vi "Word Finder.vi"() -> ()   [LabVIEW 2023]
uses:
  af6e6935-e207-d649-a71b-7505053b652b.vi
panel:
  out "msg":string
  out "words":string[](array[string])
  in  "file":path=path "Gettysburg.txt"
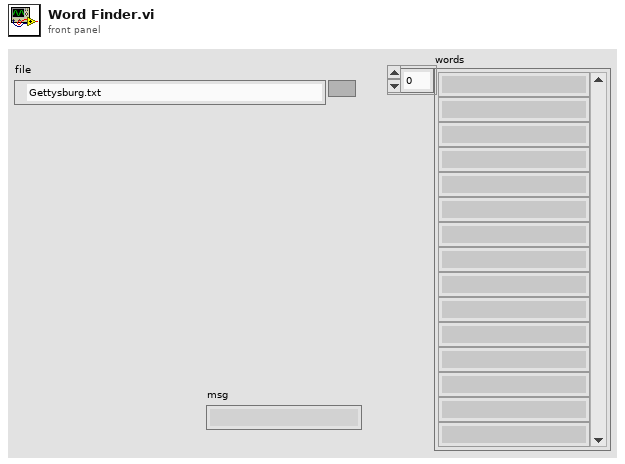
[diagram p1: front panel]
types:
  T1 = enum16{"_Quit_", "Init", "Space", "Word", "Error", "Done"}
  T2 = enum16{"_Quit_", "Init", "Space", "Word", "Error", "Done"}[]
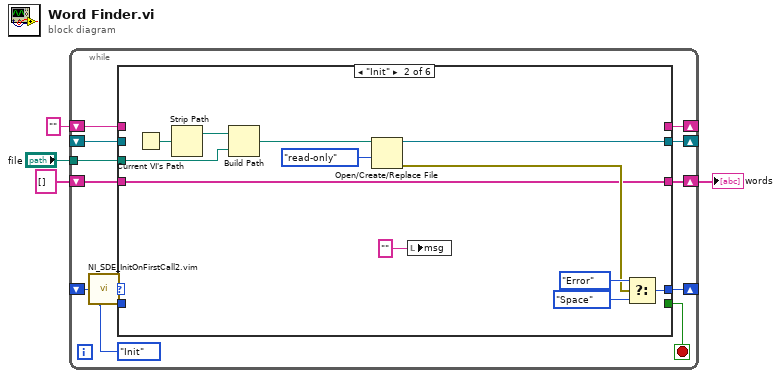
[diagram p0: block diagram]
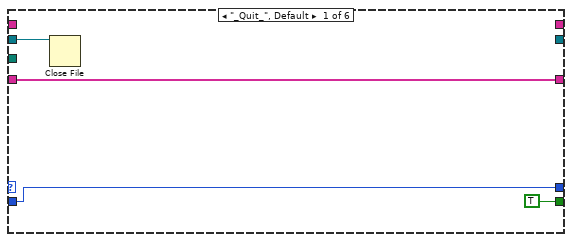
[diagram p2: hidden frame]
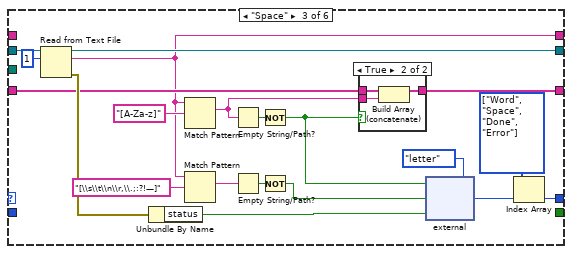
[diagram p3: hidden frame]
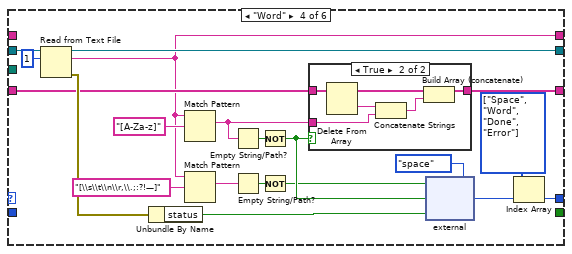
[diagram p5: hidden frame]
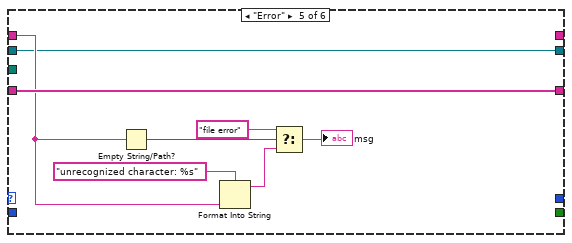
[diagram p7: hidden frame]
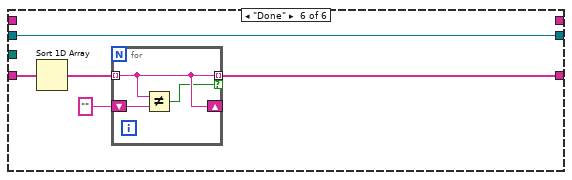
[diagram p8: hidden frame]
diagram:
  n1 = while {
    shift-right: [w12] -> w3
    shift-left: string[] [] -> [w11]
    tunnel: "file" -> [w14]
    shift-right: [w13] -> _
    shift-left: _ -> [w10]
    shift-right: [w9] -> _
    shift-left: "" -> [w8]
    shift-right: [w7] -> _
    shift-left: _ -> [w6]
    stop <- w16 stop-if-true
    w15 = T1."Init"
    n2 = call "NI_SDE_InitOnFirstCall2.vim"("input"=w6, "master enum"=w15) -> ("output enum"=w5:T1)  [unwired: 1 in]
    n3 = case shown="\"Init\"" w5 {
      tunnel: [TRUE _ _ _ _ _] -> w16
      tunnel: [w19 w31 w52 w86 _ _] -> w7
      tunnel: w15 -> [w19 _ _ _ _ _]
      tunnel: w14 -> [_ w21 _ _ _ _]
      tunnel: [_ w28 w46 w71 w104 w112] -> w13
      tunnel: [w17 w26 w35 w74 w111 w114] -> w12
      tunnel: w11 -> [w17 w26 w36 w73 w111 w116]
      tunnel: w10 -> [w18 _ w48 w72 w104 w112]
      tunnel: [_ _ w33 w67 _ _] -> w9
      tunnel: w8 -> [_ _ _ _ w107 _]
      frame "_Quit_", Default {
        n4 = Close File(refnum=w18) -> ()  [unwired: 1 in, 2 out]
      }
      frame "Init" {
        n5 = Current VI's Path() -> (path=w24:path)
        n6 = Strip Path(path=w24) -> (stripped path=w23:path)  [unwired: 1 out]
        n7 = Build Path(base path=w23, name or relative path=w21) -> (appended path=w22:path)
        n8 = Open/Create/Replace File(file path (use dialog)=w22, access (0:read/write)=enum16{"read/write", "read-only", "write-only"}."read-only") -> (refnum out=w28:refnum<file>, error out=w27:errorcluster)  [unwired: 4 in, 1 out]
        n9 = local write "msg"("" ("msg")) -> ()
        n10 = Select(t=T1."Error" ("output enum"), s=w27, f=T1."Space") -> (s? t:f=w31:T1)
      }
      frame "Space" {
        w49 = T2 [enum."Word", enum."Space", enum."Done", enum."Error"] items=["_Quit_", "Init", "Space", "Word", "Error", "Done"]
        n11 = Read from Text File(file (use dialog)=w48, count=1) -> (refnum out=w46:refnum<file>, text=w33:string, error out=w45:errorcluster)  [unwired: 2 in, 1 out]
        n12 = Unbundle By Name(w45) -> ("status"=w44:bool)
        n13 = Match Pattern(string=w33, regular expression="[A-Za-z]") -> (match substring=w34:string)  [unwired: 1 in, 3 out]
        n14 = Match Pattern(string=w33, regular expression="[\\s\\t\\n\\r,\\.;:?!—]") -> (match substring=w41:string)  [unwired: 1 in, 3 out]
        n15 = Empty String/Path?(string/path=w34) -> (empty?=w38:bool)
        n16 = Empty String/Path?(string/path=w41) -> (empty?=w39:bool)
        n17 = Not(x=w38) -> (.not. x?=w37:bool)
        n18 = Not(x=w39) -> (.not. x?=w40:bool)
        n19 = case shown="True" w37 {
          tunnel: w36 -> [w53 w56]
          tunnel: [w53 w55] -> w35
          tunnel: w34 -> [_ w54]
          frame False {
          }
          frame True {
            n20 = Build Array (concatenate)(w56, w54) -> (w55:string[])
          }
        }
        n21 = external ("First Transition")(enum16{"letter", "space", "eof", "default"}."letter", w37, w40, w44) -> (w51:enum16{"letter", "space", "eof", "default"})
        n22 = Index Array(array=w49, index=w51) -> (element=w52:T1)
      }
      frame "Word" {
        w83 = T2 [enum."Space", enum."Word", enum."Done", enum."Error"] items=["_Quit_", "Init", "Space", "Word", "Error", "Done"]
        n23 = Read from Text File(file (use dialog)=w72, count=1) -> (refnum out=w71:refnum<file>, text=w67:string, error out=w81:errorcluster)  [unwired: 2 in, 1 out]
        n24 = Unbundle By Name(w81) -> ("status"=w70:bool)
        n25 = Match Pattern(string=w67, regular expression="[A-Za-z]") -> (match substring=w75:string)  [unwired: 1 in, 3 out]
        n26 = Match Pattern(string=w67, regular expression="[\\s\\t\\n\\r,\\.;:?!—]") -> (match substring=w78:string)  [unwired: 1 in, 3 out]
        n27 = Empty String/Path?(string/path=w75) -> (empty?=w76:bool)
        n28 = Empty String/Path?(string/path=w78) -> (empty?=w77:bool)
        n29 = Not(x=w76) -> (.not. x?=w69:bool)
        n30 = Not(x=w77) -> (.not. x?=w68:bool)
        n31 = case shown="True" w69 {
          tunnel: w73 -> [w87 w92]
          tunnel: [w87 w93] -> w74
          tunnel: w75 -> [_ w89]
          frame False {
          }
          frame True {
            n32 = Delete From Array(array=w92) -> (deleted portion=w90:string, array with subset deleted=w91:string[])  [unwired: 2 in]
            n33 = Concatenate Strings(w90, w89) -> (w88:string)
            n34 = Build Array (concatenate)(w91, w88) -> (w93:string[])
          }
        }
        n35 = external ("First Transition")(enum16{"space", "letter", "eof", "default"}."space", w68, w69, w70) -> (w85:enum16{"space", "letter", "eof", "default"})
        n36 = Index Array(array=w83, index=w85) -> (element=w86:T1)
      }
      frame "Error" {
        n37 = Empty String/Path?(string/path=w107) -> (empty?=w110:bool)
        n38 = Format Into String(format string="unrecognized character: %s", w107) -> (resulting string=w105:string)  [unwired: 2 in, 1 out]
        n39 = Select(t="file error", s=w110, f=w105) -> (s? t:f=→"msg":string)
      }
      frame "Done" {
        n40 = Sort 1D Array(array=w116) -> (sorted array=w115:string[])
        n41 = for {
          tunnel: w115 -> [w119] mode=indexing
          tunnel: [w119] -> w114 mode=indexing if=w117
          shift-right: [w119] -> _
          shift-left: "" -> [w118]
          n42 = Not Equal?(x=w119, y=w118) -> (x != y?=w117:bool)
        }
      }
    }
  }
  "words" <- w3
